vi "ExSubFullBin.vi"(2 "error in (no error)":errorcluster, 3 "Camera Handle":u32) -> (0 "error out":errorcluster, 1 "Camera Handle":u32)   [LabVIEW 2010]
uses:
  GlobalExposure.vi
  GlobalFramesToStr.vi
  GlobalAcquireFocusFlag.vi
  GlobalCCDMaxDim.vi
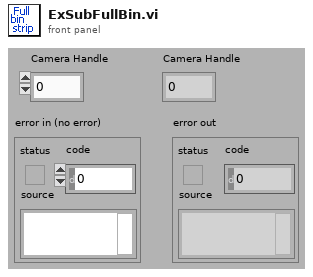
[diagram p1: front panel]
types:
  T1 = cluster{i32, "CCD Max X":u32, i32, i32, "CCD Max Y":u32, "CCD Max Y":u32}
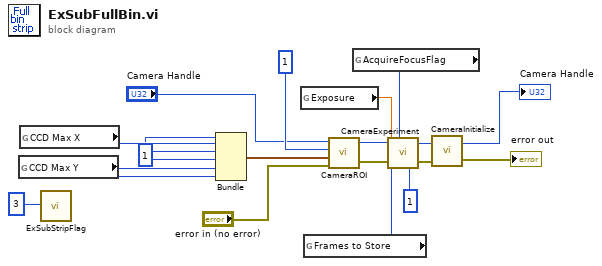
[diagram p0: block diagram]
diagram:
  w6 = 1
  n1 = global read "GlobalCCDMaxDim.vi" "CCD Max Y"() -> (w5:u32)
  n2 = global read "GlobalCCDMaxDim.vi" "CCD Max X"() -> (w10:u32)
  n3 = call "ExSubStripFlag.vi"("Binning \nUser = 1\nCenter = 2\nFull = 3"=3) -> ()
  n4 = Bundle(w6, "CCD Max X"=w10, w6, w6, "CCD Max Y"=w5, "CCD Max Y"=w5) -> (w9:T1)  [unwired: 1 in]
  n5 = global read "GlobalExposure.vi" "Exposure"() -> (w13:dbl)
  n6 = global read "GlobalFramesToStr.vi" "Frames to Store"() -> (w12:u32)
  n7 = call <userlib>:"CameraROI.vi"("error in"="error in (no error)", "ROI Params"=w9, "ROI Index"=1, "Camera Handle"="Camera Handle") -> ("error out"=w16:errorcluster, "Camera Handle"=w18:u32)
  n8 = global read "GlobalAcquireFocusFlag.vi" "AcquireFocusFlag"() -> (w11:u32)
  n9 = call <userlib>:"CameraExperiment.vi"("Number of Accumulations"=1, "Acquire / Focus Flag"=w11, "error in"=w16, "Number of Images"=w12, "Exposure (sec)"=w13, "Camera Handle"=w18) -> ("error out"=w15:errorcluster, "Camera Handle"=w17:u32)
  n10 = call <userlib>:"CameraInitialize.vi"("error in"=w15, "Camera Handle"=w17) -> ("error out"=→"error out":errorcluster, "Camera Handle"=→"Camera Handle":u32)
